vi "Servo Motor (子VI).vi"(10 "Direction":bool[](array[boolean])=[FALSE, FALSE, FALSE, FALSE, FALSE, FALSE], 11 "Custom FPGA Reference Out":refnum<k20>) -> ()   [LabVIEW 2017, in "年前程序.lvlib"]
uses:
  <vilib>/Utility/error.llb/Error Cluster From Error Code.vi
  <vilib>/rvi/errors/niLvFpgaAdjustHostInterfaceError.vi
  <vilib>/rvi/interface/nirviReadWriteControl/nirviReadWriteControl.xnode
  NiFpgaLv.dll
  <vilib>/rvi/interface/Simulation/niFpgaSimulationCallBeginRW.vi
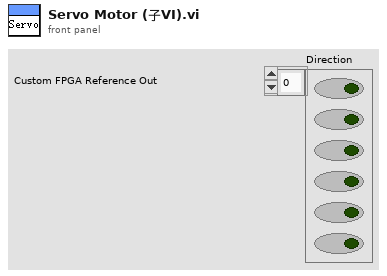
[diagram p1: front panel]
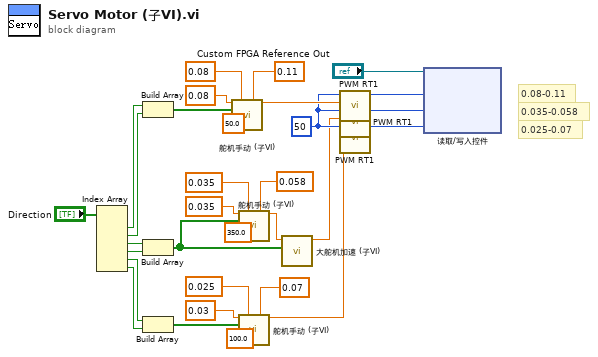
[diagram p0: block diagram]
diagram:
  w4 = u16 50 ("频率")
  # "0.025-0.07"
  # "0.035-0.058"
  # "0.08-0.11"
  n1 = Index Array(array="Direction") -> (element #1=w24:bool, element #2=w25:bool, element #3=w26:bool, element #4=w28:bool, element #5=w27:bool, element #6=w29:bool)  [unwired: 6 in]
  n2 = Build Array(w24, w25) -> (w30:bool[])
  n3 = Build Array(w26, w28) -> (w14:bool[])
  n4 = Build Array(w27, w29) -> (w31:bool[])
  n5 = call "舵机手动 (子VI).vi"("初始化"=0.08, "下限"=0.08, "上限"=0.11, "方向"=w30, "加速率"=50.0 ("加速率 2")) -> ("PWM输出"=w5:dbl)  [unwired: 10 in]
  n6 = call "舵机手动 (子VI).vi"("初始化"=0.035, "下限"=0.035, "上限"=0.058, "方向"=w14, "加速率"=350.0) -> ("PWM输出"=w12:dbl)  [unwired: 10 in]
  n7 = call "舵机手动 (子VI).vi"("初始化"=0.03, "下限"=0.025, "上限"=0.07, "方向"=w31, "加速率"=100.0 ("加速率 3")) -> ("PWM输出"=w6:dbl)  [unwired: 10 in]
  n8 = call "大舵机加速 (子VI).vi"("数组"=w14, "PWM输入"=w12) -> ("PWM输出 2"=w3:dbl)  [unwired: 9 in]
  n9 = call "PWM RT1.vi"("占空比"=w5, "频率"=w4) -> ("PWM FT"=w7:u32)  [unwired: 9 in]
  n10 = call "PWM RT1.vi"("占空比"=w3, "频率"=w4) -> ("PWM FT"=w1:u32)  [unwired: 9 in]
  n11 = call "PWM RT1.vi"("占空比"=w6, "频率"=w4) -> ("PWM FT"=w2:u32)  [unwired: 9 in]
  n12 = xnode "读取/写入控件"("FPGA VI引用输入"="Custom FPGA Reference Out", "PWM FT 5"=w7, "PWM FT 6"=w1, "PWM FT 7"=w2) -> ()  [unwired: 1 in, 2 out]
